vi "SwitchRT.vi"(8 "error in (no error)":errorcluster) -> (0 "error out":errorcluster, 3 "RemoteState":T1)   [LabVIEW 2016]
uses:
  controls/SwitchStates.ctl
  controls/RT-Variables.lvlib
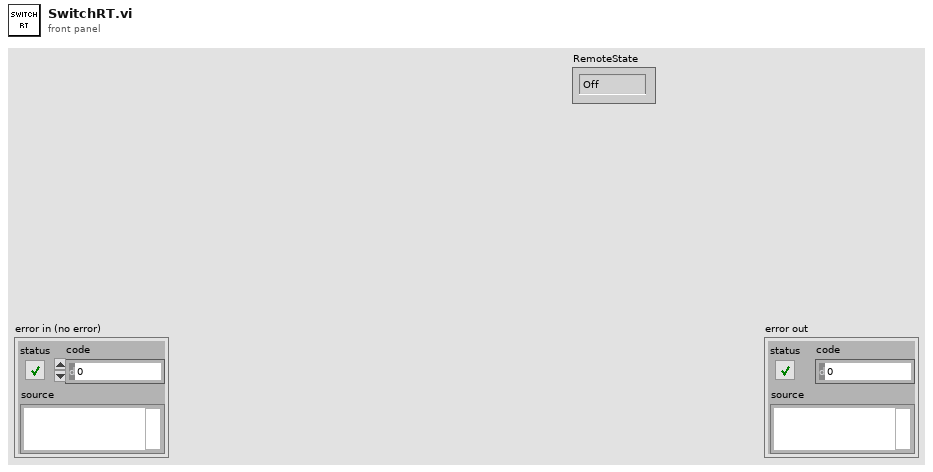
[diagram p1: front panel]
types:
  T1 = typedef "RT-Variables.lvlib/SwitchStates.ctl" = enum16{"Off", "Local", "Remote"}
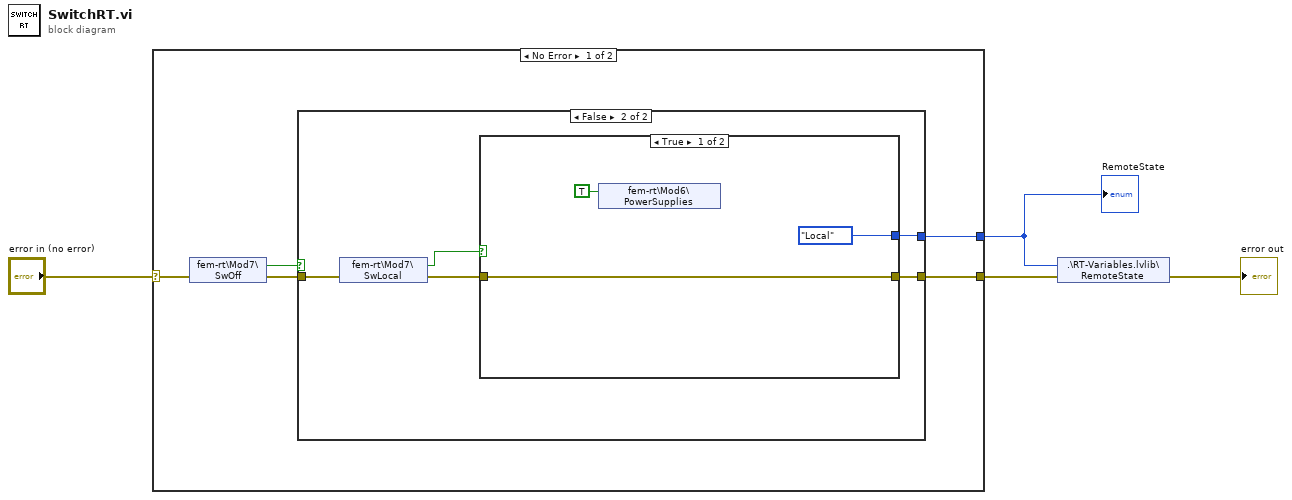
[diagram p0: block diagram]
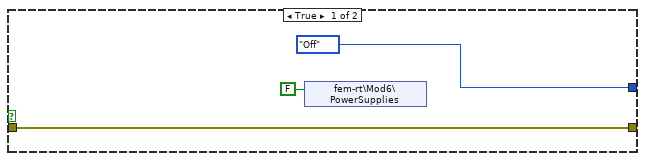
[diagram p2: hidden frame]
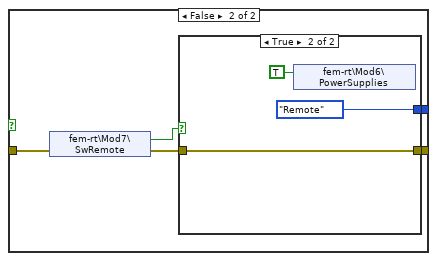
[diagram p3: hidden frame]
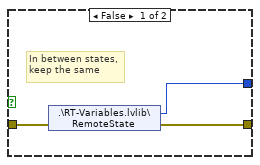
[diagram p4: hidden frame]
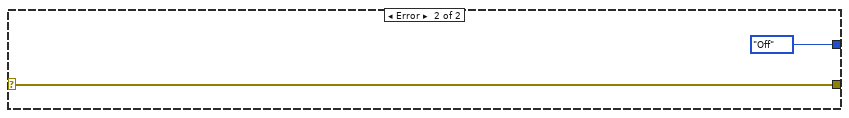
[diagram p5: hidden frame]
diagram:
  n1 = case shown="No Error" "error in (no error)" {
    selector: "error in (no error)" -> [w7 w33]
    tunnel: [w8 w33] -> w3
    tunnel: [w5 SwitchStates."Off" ("RemoteState")] -> w1
    frame No Error {
      n2 = shared-variable "fem-rt\\Mod7\\SwOff"(error in=w7) -> (w6:bool, error out=w9:errorcluster)
      n3 = case shown="False" w6 {
        tunnel: w9 -> [w11 w17]
        tunnel: [w11 w15] -> w8
        tunnel: [SwitchStates."Off" ("RemoteState") w13] -> w5
        frame True {
          n4 = shared-variable "fem-rt\\Mod6\\PowerSupplies"(FALSE ("DO0")) -> ()  [unwired: 1 in, 1 out]
        }
        frame False {
          n5 = shared-variable "fem-rt\\Mod7\\SwLocal"(error in=w17) -> (w14:bool, error out=w16:errorcluster)
          n6 = case shown="True" w14 {
            tunnel: w16 -> [w20 w25]
            tunnel: [w20 w23] -> w15
            tunnel: [SwitchStates."Local" ("RemoteState") w21] -> w13
            frame True {
              n7 = shared-variable "fem-rt\\Mod6\\PowerSupplies"(TRUE ("DO0")) -> ()  [unwired: 1 in, 1 out]
            }
            frame False {
              n8 = shared-variable "fem-rt\\Mod7\\SwRemote"(error in=w25) -> (w22:bool, error out=w24:errorcluster)
              n9 = case shown="True" w22 {
                tunnel: w24 -> [w27 w31]
                tunnel: [w26 w31] -> w23
                tunnel: [w28 SwitchStates."Remote" ("RemoteState")] -> w21
                frame False {
                  # "In between states,\nkeep the same"
                  n10 = shared-variable ".\\RT-Variables.lvlib\\RemoteState"(error in=w27) -> (w28:T1, error out=w26:errorcluster)
                }
                frame True {
                  n11 = shared-variable "fem-rt\\Mod6\\PowerSupplies"(TRUE ("DO0")) -> ()  [unwired: 1 in, 1 out]
                }
              }
            }
          }
        }
      }
    }
    frame Error {
    }
  }
  "RemoteState" <- w1
  n12 = shared-variable ".\\RT-Variables.lvlib\\RemoteState"(w1, error in=w3) -> (error out=→"error out":errorcluster)
